vi "Save CAN Frame to TDMS v2.vi"(0 "tdms file in":refnum<k34>, 1 "group name in":string, 2 "CAN Frame":u32[](array[numeric]), 3 "error in":errorcluster) -> (7 "tdms file out":refnum<k34>, 8 "group name out":string, 10 "error out":errorcluster)   [LabVIEW 2016]
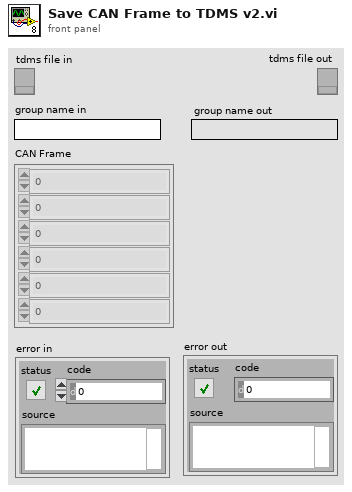
[diagram p1: front panel]
types:
  T1 = cluster{"CAN Frame[0]":u32, "CAN Frame[1]":u32, "CAN Frame[2]":u32, "CAN Frame[3]":u32, "CAN Frame[4]":u32, "CAN Frame[5]":u32}
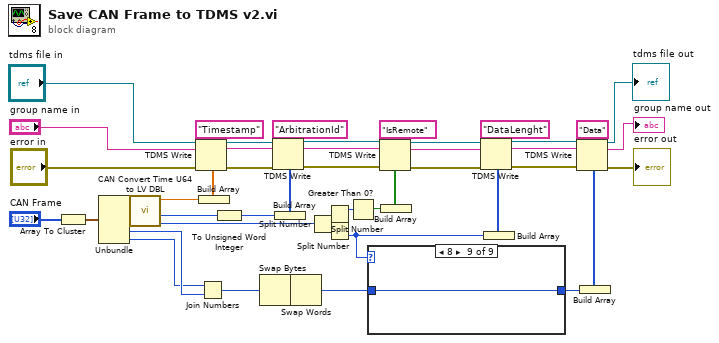
[diagram p0: block diagram]
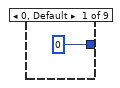
[diagram p2: hidden frame]
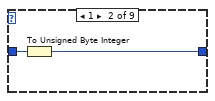
[diagram p3: hidden frame]
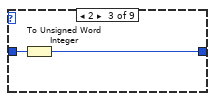
[diagram p4: hidden frame]
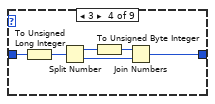
[diagram p5: hidden frame]
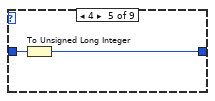
[diagram p6: hidden frame]
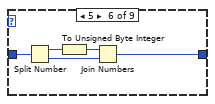
[diagram p7: hidden frame]
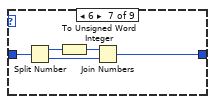
[diagram p8: hidden frame]
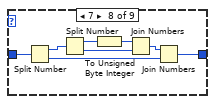
[diagram p9: hidden frame]
diagram:
  n1 = Array To Cluster(array="CAN Frame") -> (cluster=w43:T1)
  n2 = Unbundle(w43) -> ("CAN Frame[0]"=w42:u32, "CAN Frame[1]"=w41:u32, "CAN Frame[2]"=w3:u32, "CAN Frame[3]"=w45:u32, "CAN Frame[4]"=w30:u32, "CAN Frame[5]"=w29:u32)
  n3 = call <vilib>:"CAN Convert Time U64 to LV DBL.vi"("Time U64 LowPart"=w41, "Time U64 HighPart"=w42) -> ("Time LV DBL"=w1:dbl)  [unwired: 3 in]
  n4 = Join Numbers(hi=w29, lo=w30) -> ((hi.lo)=w28:u64)
  n5 = Build Array(w1) -> (w40:dbl[])
  n6 = TDMS Write(0:"tdms file in", 5:"group name in", 7:"Timestamp" ("String"), 9:w40, 11:"error in") -> (4:w23:refnum<k34>, 6:w22:string, 15:w21:errorcluster)  [unwired: 1 in, 1 out]
  n7 = To Unsigned Word Integer(number=w3) -> (unsigned 16bit integer=w4:u16)
  n8 = Swap Bytes(anything=w28) -> (byte swapped=w31:u64)
  n9 = Build Array(w4) -> (w12:u16[])
  n10 = TDMS Write(0:w23, 5:w22, 7:"ArbitrationId", 9:w12, 11:w21) -> (4:w20:refnum<k34>, 6:w11:string, 15:w19:errorcluster)  [unwired: 1 in, 1 out]
  n11 = Swap Words(1:w31) -> (0:w27:u64)
  n12 = Split Number(x=w45) -> (hi(x)=w46:u16, lo(x)=w47:u16)
  n13 = Split Number(x=w46) -> (hi(x)=w39:u8)  [unwired: 1 out]
  n14 = Split Number(x=w47) -> (lo(x)=w14:u8)  [unwired: 1 out]
  n15 = Greater Than 0?(x=w39) -> (x > 0?=w2:bool)
  n16 = case shown="8" w14 {
    tunnel: w27 -> [_ w50 w52 w58 w60 w65 w67 w71 w79]
    tunnel: [0 w49 w51 w53 w59 w61 w66 w72 w79] -> w26
    frame 0, Default {
    }
    frame 1 {
      n17 = To Unsigned Byte Integer(number=w50) -> (unsigned 8bit integer=w49:u8)
    }
    frame 2 {
      n18 = To Unsigned Word Integer(number=w52) -> (unsigned 16bit integer=w51:u16)
    }
    frame 3 {
      n19 = To Unsigned Long Integer(number=w58) -> (unsigned 32bit integer=w57:u32)
      n20 = Split Number(x=w57) -> (hi(x)=w56:u16, lo(x)=w54:u16)
      n21 = To Unsigned Byte Integer(number=w56) -> (unsigned 8bit integer=w55:u8)
      n22 = Join Numbers(hi=w55, lo=w54) -> ((hi.lo)=w53:u32)
    }
    frame 4 {
      n23 = To Unsigned Long Integer(number=w60) -> (unsigned 32bit integer=w59:u32)
    }
    frame 5 {
      n24 = Split Number(x=w65) -> (hi(x)=w64:u32, lo(x)=w62:u32)
      n25 = To Unsigned Byte Integer(number=w64) -> (unsigned 8bit integer=w63:u8)
      n26 = Join Numbers(hi=w63, lo=w62) -> ((hi.lo)=w61:u64)
    }
    frame 6 {
      n27 = Split Number(x=w67) -> (hi(x)=w70:u32, lo(x)=w68:u32)
      n28 = To Unsigned Word Integer(number=w70) -> (unsigned 16bit integer=w69:u16)
      n29 = Join Numbers(hi=w69, lo=w68) -> ((hi.lo)=w66:u64)
    }
    frame 7 {
      n30 = Split Number(x=w71) -> (hi(x)=w76:u32, lo(x)=w77:u32)
      n31 = Split Number(x=w76) -> (hi(x)=w73:u16, lo(x)=w78:u16)
      n32 = To Unsigned Byte Integer(number=w73) -> (unsigned 8bit integer=w74:u8)
      n33 = Join Numbers(hi=w74, lo=w78) -> ((hi.lo)=w75:u32)
      n34 = Join Numbers(hi=w75, lo=w77) -> ((hi.lo)=w72:u64)
    }
    frame 8 {
    }
  }
  n35 = Build Array(w2) -> (w38:bool[])
  n36 = TDMS Write(0:w20, 5:w11, 7:"IsRemote" ("String"), 9:w38, 11:w19) -> (4:w18:refnum<k34>, 6:w10:string, 15:w17:errorcluster)  [unwired: 1 in, 1 out]
  n37 = Build Array(w14) -> (w13:u8[])
  n38 = TDMS Write(0:w18, 5:w10, 7:"DataLenght", 9:w13, 11:w17) -> (4:w16:refnum<k34>, 6:w9:string, 15:w15:errorcluster)  [unwired: 1 in, 1 out]
  n39 = Build Array(w26) -> (w25:u64[])
  n40 = TDMS Write(0:w16, 5:w9, 7:"Data" ("String"), 9:w25, 11:w15) -> (4:→"tdms file out":refnum<k34>, 6:→"group name out":string, 15:→"error out":errorcluster)  [unwired: 1 in, 1 out]
